vi "Compile Datalog Array sub_VI.vi"(2 "XY Cluster":T1={"X Data"={"Complete?"=FALSE, "Motor Params"={"Duty %"=0.0, "X Freq"=0.0, "FWD/RVS"=FALSE}, "SP"={"Accel"=0.0, "Decel"=0.0, "Speed"=0.0}, "State"=enum."Stop", "Input"={"Coord"=0.0, "Tol"=0.0, "Accel"=0.0, "Decel"=0.0, "Max Speed"=0.0}, "Path"={"V plan"=[], "V actual"=[], "S actual"=[], "a actual"=[], "Profile"=enum."Triangular", "Decel Dist"=0.0, "Accel Dist"=0.0, "Cruise V"=0.0, "Cruise Dist"=0.0}, "PID"={"Kc"=0.0, "Ti"=0.0, "Td"=0.0}, "Motion"={"Speed"=0.0, "Dist"=0.0, "Acceleration"=0.0, "Dist to target"=0.0}}, "Y Data"={"Complete?"=FALSE, "Motor Params"={"Duty %"=0.0, "Freq"=0.0, "FWD/RVS"=FALSE}, "SP"={"Y Accel"=0.0, "Y Decel"=0.0, "Speed"=0.0}, "State"=enum."Stop", "Input"={"Coord"=0.0, "Tol"=0.0, "Accel"=0.0, "Decel"=0.0, "Max Speed"=0.0}, "Path"={"V plan"=[], "V actual"=[], "S actual"=[], "a actual"=[], " Profile"=enum."Triangular", "Decel Dist"=0.0, "Accel Dist"=0.0, "Cruise V"=0.0, "Cruise Dist"=0.0}, "PID"={"Kc"=0.0, "Ti"=0.0, "Td"=0.0}, "Motion"={"Speed"=0.0, "Dist"=0.0, "Acceleration"=0.0, "Dist to target"=0.0}}, "Timing"={"Runtime"=0.0, "Loop time"=0.0, "Loop iter"=0, "Tick"=0.0}, "stop"=FALSE} {"Y Data"."Input"."Tol" min=0.0; "X Data"."Input"."Tol" min=0.0}, 3 "Initialised Array":string[][](array[string])) -> (0 "Data Array":string[][](array[string]))   [LabVIEW 2017]
uses:
  XY Cluster.ctl
  Motor Status Enum.ctl
  Motion Type Def.ctl
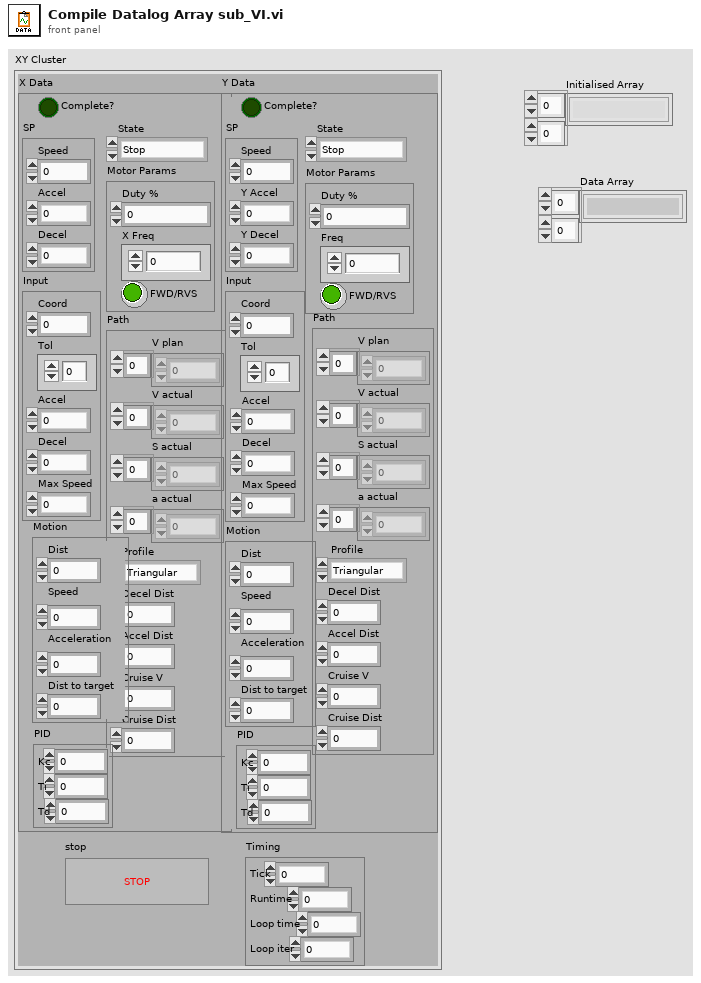
[diagram p1: front panel]
types:
  T1 = typedef "XY Cluster.ctl" = cluster{"X Data":cluster{"Complete?":bool, "Motor Params":cluster{"Duty %":dbl, "X Freq":dbl, "FWD/RVS":bool}, "SP":cluster{"Accel":dbl, "Decel":dbl, "Speed":dbl}, "State":T2, "Input":cluster{"Coord":dbl, "Tol":dbl, "Accel":dbl, "Decel":dbl, "Max Speed":dbl}, "Path":cluster{"V plan":dbl[], "V actual":dbl[], "S actual":dbl[], "a actual":dbl[], "Profile":T3, "Decel Dist":dbl, "Accel Dist":dbl, "Cruise V":dbl, "Cruise Dist":dbl}, "PID":cluster{"Kc":dbl, "Ti":dbl, "Td":dbl}, "Motion":cluster{"Speed":dbl, "Dist":dbl, "Acceleration":dbl, "Dist to target":dbl}}, "Y Data":cluster{"Complete?":bool, "Motor Params":cluster{"Duty %":dbl, "Freq":dbl, "FWD/RVS":bool}, "SP":cluster{"Y Accel":dbl, "Y Decel":dbl, "Speed":dbl}, "State":T2, "Input":cluster{"Coord":dbl, "Tol":dbl, "Accel":dbl, "Decel":dbl, "Max Speed":dbl}, "Path":cluster{"V plan":dbl[], "V actual":dbl[], "S actual":dbl[], "a actual":dbl[], " Profile":T3, "Decel Dist":dbl, "Accel Dist":dbl, "Cruise V":dbl, "Cruise Dist":dbl}, "PID":cluster{"Kc":dbl, "Ti":dbl, "Td":dbl}, "Motion":cluster{"Speed":dbl, "Dist":dbl, "Acceleration":dbl, "Dist to target":dbl}}, "Timing":cluster{"Runtime":dbl, "Loop time":dbl, "Loop iter":i32, "Tick":dbl}, "stop":bool}
  T2 = typedef "Motor Status Enum.ctl" = enum16{"Update I/O", "Stop", "Steady Speed", "Accelerate", "Decelerate", "Drive Motor"}
  T3 = typedef "Motion Type Def.ctl" = enum16{"Trapezodial", "Triangular"}
  T4 = cluster{"Complete?":bool, "Motor Params":cluster{"Duty %":dbl, "X Freq":dbl, "FWD/RVS":bool}, "SP":cluster{"Accel":dbl, "Decel":dbl, "Speed":dbl}, "State":T2, "Input":cluster{"Coord":dbl, "Tol":dbl, "Accel":dbl, "Decel":dbl, "Max Speed":dbl}, "Path":cluster{"V plan":dbl[], "V actual":dbl[], "S actual":dbl[], "a actual":dbl[], "Profile":T3, "Decel Dist":dbl, "Accel Dist":dbl, "Cruise V":dbl, "Cruise Dist":dbl}, "PID":cluster{"Kc":dbl, "Ti":dbl, "Td":dbl}, "Motion":cluster{"Speed":dbl, "Dist":dbl, "Acceleration":dbl, "Dist to target":dbl}}
  T5 = cluster{"Complete?":bool, "Motor Params":cluster{"Duty %":dbl, "Freq":dbl, "FWD/RVS":bool}, "SP":cluster{"Y Accel":dbl, "Y Decel":dbl, "Speed":dbl}, "State":T2, "Input":cluster{"Coord":dbl, "Tol":dbl, "Accel":dbl, "Decel":dbl, "Max Speed":dbl}, "Path":cluster{"V plan":dbl[], "V actual":dbl[], "S actual":dbl[], "a actual":dbl[], " Profile":T3, "Decel Dist":dbl, "Accel Dist":dbl, "Cruise V":dbl, "Cruise Dist":dbl}, "PID":cluster{"Kc":dbl, "Ti":dbl, "Td":dbl}, "Motion":cluster{"Speed":dbl, "Dist":dbl, "Acceleration":dbl, "Dist to target":dbl}}
  T6 = cluster{"Runtime":dbl, "Loop time":dbl, "Loop iter":i32}
  T7 = cluster{i16, i16, "Duty %":dbl, "X Freq":dbl, "Speed":dbl, "Speed":dbl, "Dist":dbl, "Acceleration":dbl, "State":T2, "Coord":dbl, "Dist to target":dbl, "Tol":dbl, "Profile":T3, "Accel Dist":dbl, "Cruise Dist":dbl, "Decel Dist":dbl, "Cruise V":dbl, "Kc":dbl, "Ti":dbl, "Td":dbl}
  T8 = cluster{i16, i16, "Duty %":dbl, "Freq":dbl, "Speed":dbl, "Speed":dbl, "Dist":dbl, "Acceleration":dbl, "State":T2, "Coord":dbl, "Dist to target":dbl, "Tol":dbl, " Profile":T3, "Accel Dist":dbl, "Cruise Dist":dbl, "Decel Dist":dbl, "Cruise V":dbl, "Kc":dbl, "Ti":dbl, "Td":dbl}
  T9 = cluster{"Runtime":string, "Loop time":string, "Loop iter":string}
  T10 = cluster{string, string, "Duty %":string, "X Freq":string, "Speed":string, "Speed":string, "Dist":string, "Acceleration":string, string, "Coord":string, "Dist to target":string, "Tol":string, string, "Accel Dist":string, "Cruise Dist":string, "Decel Dist":string, "Cruise V":string, "Kc":string, "Ti":string, "Td":string}
  T11 = cluster{string, string, "Duty %":string, "Freq":string, "Speed":string, "Speed":string, "Dist":string, "Acceleration":string, string, "Coord":string, "Dist to target":string, "Tol":string, string, "Accel Dist":string, "Cruise Dist":string, "Decel Dist":string, "Cruise V":string, "Kc":string, "Ti":string, "Td":string}
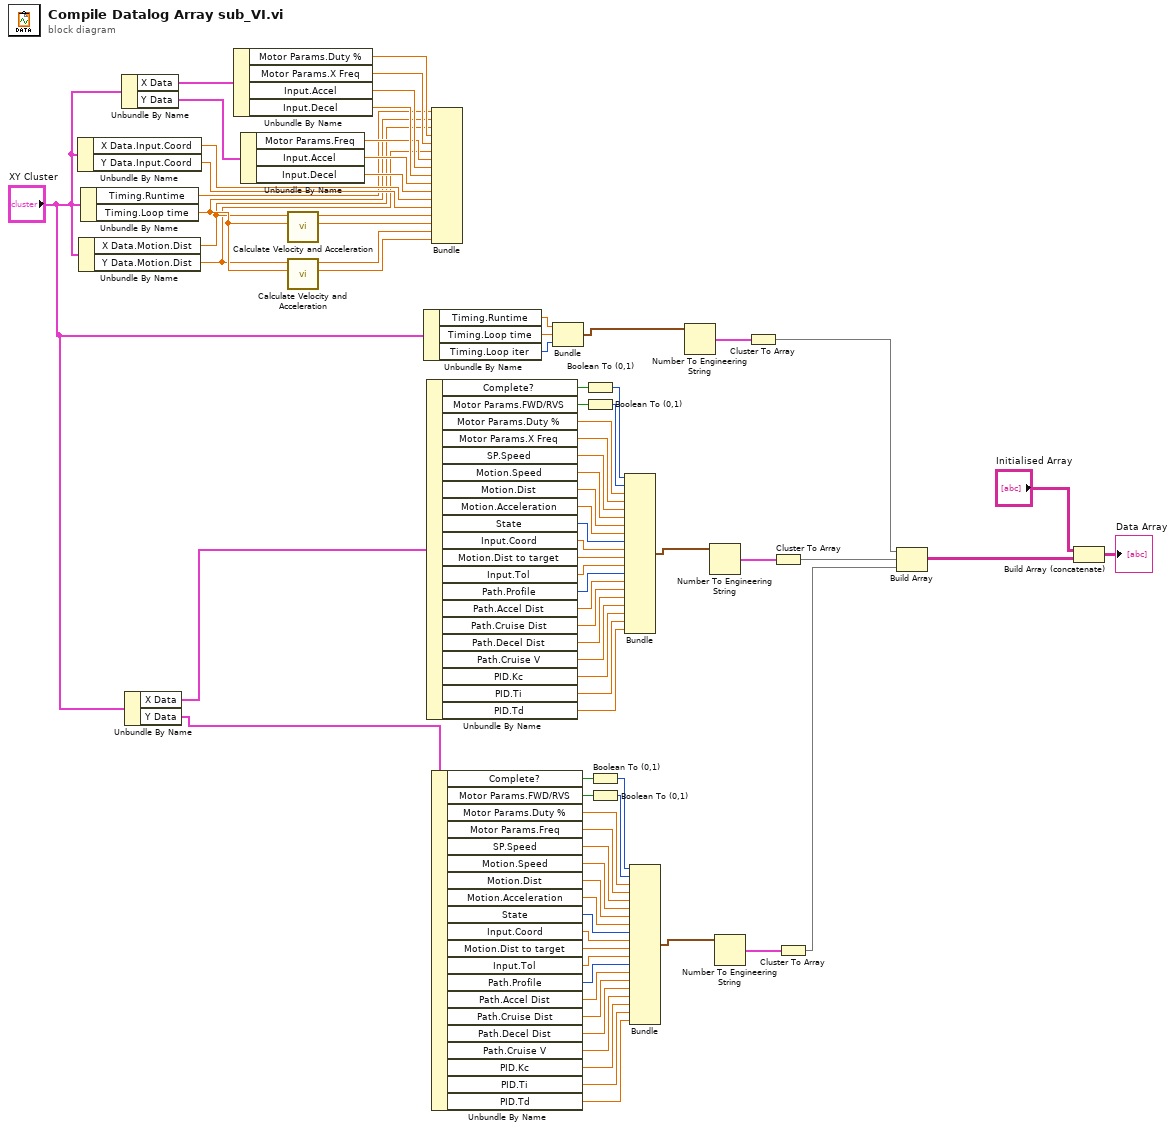
[diagram p0: block diagram]
diagram:
  n1 = Unbundle By Name("XY Cluster") -> ("X Data.Input.Coord"=w66:dbl, "Y Data.Input.Coord"=w65:dbl)
  n2 = Unbundle By Name("XY Cluster") -> ("X Data.Motion.Dist"=w62:dbl, "Y Data.Motion.Dist"=w61:dbl)
  n3 = Unbundle By Name("XY Cluster") -> ("Timing.Runtime"=w64:dbl, "Timing.Loop time"=w63:dbl)
  n4 = Unbundle By Name("XY Cluster") -> ("X Data"=w71:T4, "Y Data"=w70:T5)
  n5 = Unbundle By Name("XY Cluster") -> ("X Data"=w56:T4, "Y Data"=w3:T5)
  n6 = Unbundle By Name(w71) -> ("Motor Params.Duty %"=w75:dbl, "Motor Params.X Freq"=w74:dbl, "Input.Accel"=w73:dbl, "Input.Decel"=w72:dbl)
  n7 = Unbundle By Name(w70) -> ("Motor Params.Freq"=w69:dbl, "Input.Accel"=w68:dbl, "Input.Decel"=w67:dbl)
  n8 = call "Calculate Velocity and Acceleration.vi"("Loop Runtime (s)"=w63, "Displacement (mm)"=w62) -> ("Acceleration (mm/s^2)"=w78:dbl, "Velocity (mm/s)"=w77:dbl)  [unwired: 8 in]
  n9 = call "Calculate Velocity and Acceleration.vi"("Loop Runtime (s)"=w63, "Displacement (mm)"=w61) -> ("Acceleration (mm/s^2)"=w80:dbl, "Velocity (mm/s)"=w79:dbl)  [unwired: 8 in]
  n10 = Unbundle By Name("XY Cluster") -> ("Timing.Runtime"=w60:dbl, "Timing.Loop time"=w59:dbl, "Timing.Loop iter"=w58:i32)
  n11 = Unbundle By Name(w56) -> ("Complete?"=w55:bool, "Motor Params.FWD/RVS"=w54:bool, "Motor Params.Duty %"=w53:dbl, "Motor Params.X Freq"=w52:dbl, "SP.Speed"=w51:dbl, "Motion.Speed"=w50:dbl, "Motion.Dist"=w49:dbl, "Motion.Acceleration"=w48:dbl, "State"=w47:T2, "Input.Coord"=w46:dbl, "Motion.Dist to target"=w45:dbl, "Input.Tol"=w44:dbl, "Path.Profile"=w43:T3, "Path.Accel Dist"=w42:dbl, "Path.Cruise Dist"=w41:dbl, "Path.Decel Dist"=w40:dbl, "Path.Cruise V"=w39:dbl, "PID.Kc"=w38:dbl, "PID.Ti"=w37:dbl, "PID.Td"=w36:dbl)
  n12 = Bundle("Runtime"=w64, "Loop time"=w63, "Dist"=w62, "Duty %"=w75, "X Freq"=w74, "Dist"=w61, "Freq"=w69, "Accel"=w73, "Decel"=w72, "Accel"=w68, "Decel"=w67, "Coord"=w66, "Coord"=w65, "Velocity (mm/s)"=w77, "Acceleration (mm/s^2)"=w78, "Velocity (mm/s)"=w79, "Acceleration (mm/s^2)"=w80) -> ()  [unwired: 1 in, 1 out]
  n13 = Unbundle By Name(w3) -> ("Complete?"=w27:bool, "Motor Params.FWD/RVS"=w26:bool, "Motor Params.Duty %"=w25:dbl, "Motor Params.Freq"=w24:dbl, "SP.Speed"=w23:dbl, "Motion.Speed"=w22:dbl, "Motion.Dist"=w21:dbl, "Motion.Acceleration"=w20:dbl, "State"=w19:T2, "Input.Coord"=w18:dbl, "Motion.Dist to target"=w17:dbl, "Input.Tol"=w16:dbl, "Path.Profile"=w15:T3, "Path.Accel Dist"=w14:dbl, "Path.Cruise Dist"=w13:dbl, "Path.Decel Dist"=w12:dbl, "Path.Cruise V"=w11:dbl, "PID.Kc"=w10:dbl, "PID.Ti"=w9:dbl, "PID.Td"=w8:dbl)
  n14 = Bundle("Runtime"=w60, "Loop time"=w59, "Loop iter"=w58) -> (w35:T6)  [unwired: 1 in]
  n15 = Boolean To (0,1)(Boolean=w55) -> (0, 1=w31:i16)
  n16 = Boolean To (0,1)(Boolean=w54) -> (0, 1=w30:i16)
  n17 = Boolean To (0,1)(Boolean=w27) -> (0, 1=w5:i16)
  n18 = Boolean To (0,1)(Boolean=w26) -> (0, 1=w4:i16)
  n19 = Bundle(w31, w30, "Duty %"=w53, "X Freq"=w52, "Speed"=w51, "Speed"=w50, "Dist"=w49, "Acceleration"=w48, "State"=w47, "Coord"=w46, "Dist to target"=w45, "Tol"=w44, "Profile"=w43, "Accel Dist"=w42, "Cruise Dist"=w41, "Decel Dist"=w40, "Cruise V"=w39, "Kc"=w38, "Ti"=w37, "Td"=w36) -> (w32:T7)  [unwired: 1 in]
  n20 = Bundle(w5, w4, "Duty %"=w25, "Freq"=w24, "Speed"=w23, "Speed"=w22, "Dist"=w21, "Acceleration"=w20, "State"=w19, "Coord"=w18, "Dist to target"=w17, "Tol"=w16, "Profile"=w15, "Accel Dist"=w14, "Cruise Dist"=w13, "Decel Dist"=w12, "Cruise V"=w11, "Kc"=w10, "Ti"=w9, "Td"=w8) -> (w6:T8)  [unwired: 1 in]
  n21 = Number To Engineering String(4:w35) -> (0:w34:T9)  [unwired: 3 in]
  n22 = Number To Engineering String(4:w32) -> (0:w33:T10)  [unwired: 3 in]
  n23 = Number To Engineering String(4:w6) -> (0:w7:T11)  [unwired: 3 in]
  n24 = Cluster To Array(cluster=w34) -> (array=w29:string[])
  n25 = Cluster To Array(cluster=w33) -> (array=w28:string[])
  n26 = Cluster To Array(cluster=w7) -> (array=w2:string[])
  n27 = Build Array(w29, w28, w2) -> (w1:string[][])
  n28 = Build Array (concatenate)("Initialised Array", w1) -> (→"Data Array":string[][])
